vi "Format_Key_Value.vi"(11 "value":string) -> (2 "key value":u32[](array[numeric]) format="%x", 3 "Array":string[](array[string]))   [LabVIEW 2023, in "LP_CRC.lvlib"]
uses:
  LP_CRC.lvlib
  <vilib>/Utility/error.llb/Trim Whitespace One-Sided.vi
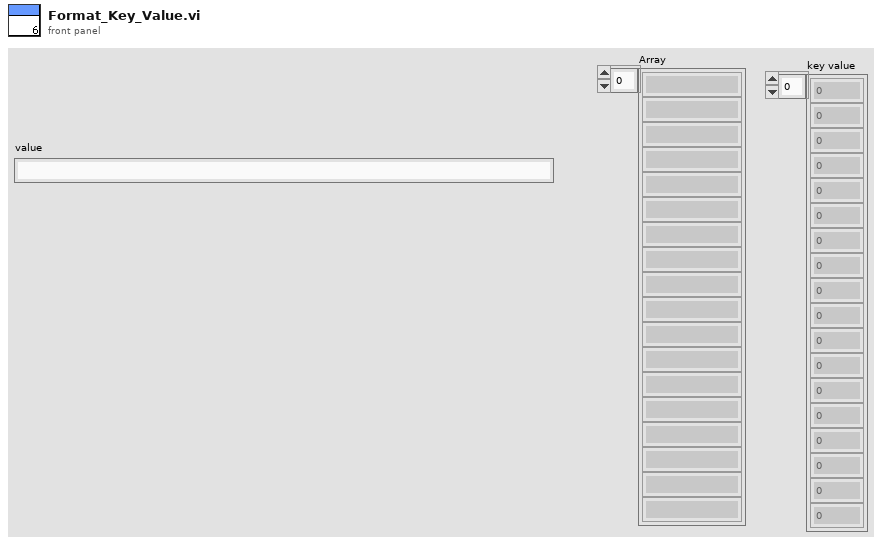
[diagram p1: front panel]
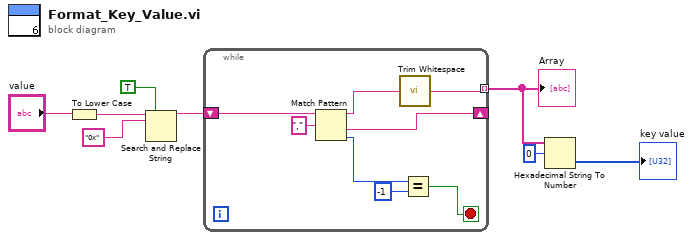
[diagram p0: block diagram]
diagram:
  n1 = To Lower Case(string="value") -> (all lower case string=w5:string)
  n2 = Search and Replace String(replace all?=TRUE ("replace all? (F)"), input string=w5, search string="0x") -> (result string=w3:string)  [unwired: 5 in, 3 out]
  n3 = while {
    shift-right: [w14] -> _
    shift-left: w3 -> [w16]
    tunnel: [w9] -> w8 mode=indexing
    stop <- w12 stop-if-true
    n4 = Match Pattern(string=w16, regular expression=",") -> (before substring=w10:string, after substring=w14:string, offset past match=w15:i32)  [unwired: 1 in, 1 out]
    n5 = call <vilib>:"Trim Whitespace.vi"("string"=w10) -> ("trimmed string"=w9:string)  [unwired: 1 in]
    n6 = Equal?(x=w15, y=-1) -> (x = y?=w12:bool)
  }
  "Array" <- w8
  n7 = Hexadecimal String To Number(string=w8, offset=0) -> (number=→"key value":u32[])  [unwired: 1 in, 1 out]
